vi "7_pressures to UVW.vi"(2 "error in (no error)":errorcluster, 3 "wait until completion?":bool=TRUE) -> (0 "error out":errorcluster)   [LabVIEW 2017]
panel:
  out "Time(s)":dbl
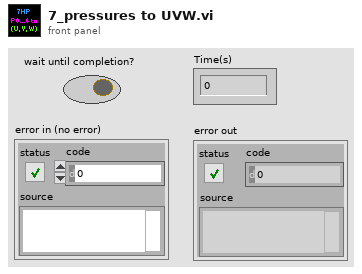
[diagram p1: front panel]
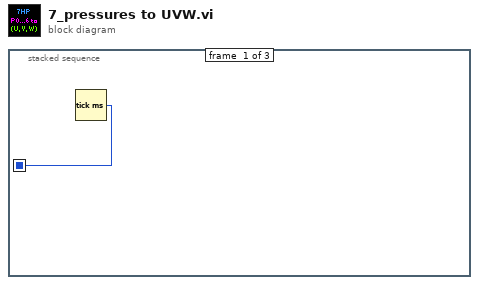
[diagram p0: block diagram]
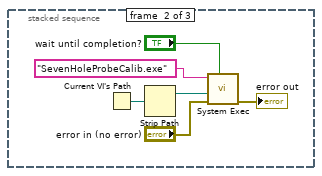
[diagram p2: hidden frame]
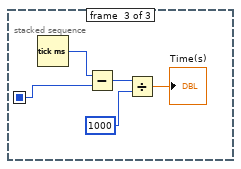
[diagram p3: hidden frame]
diagram:
  n1 = stacked-sequence {
    seq-local: [w1 _ _] -> [_ _ w11]
    frame #0 {
      n2 = Tick Count (ms)() -> (millisecond timer value=w1:u32)
    }
    frame #1 {
      n3 = Current VI's Path() -> (path=w4:path)
      n4 = Strip Path(path=w4) -> (stripped path=w3:path)  [unwired: 1 out]
      n5 = call <vilib>:"System Exec.vi"("wait until completion? (T)"="wait until completion?", "error in (no error)"="error in (no error)", "working directory"=w3, "command line"="SevenHoleProbeCalib.exe") -> ("error out"=→"error out":errorcluster)  [unwired: 4 in, 3 out]
    }
    frame #2 {
      n6 = Tick Count (ms)() -> (millisecond timer value=w12:u32)
      n7 = Subtract(x=w12, y=w11) -> (x-y=w10:u32)
      n8 = Divide(x=w10, y=u32 1000) -> (x/y=→"Time(s)":dbl)
    }
  }
